vi "Request Events.vi"(8 "error in (no error)":errorcluster, 11 "VolatusAPI in":refnum<class "VolatusAPI.lvclass">) -> (0 "error out":errorcluster, 2 "Events":T1[](array[typedef]), 3 "VolatusAPI out":refnum<class "VolatusAPI.lvclass">)   [LabVIEW 2020, in "Volatus.lvlib" / "VolatusAPI.lvclass"]
uses:
  VolatusAPI.lvclass
  VolatusAPI.lvclass/VolatusAPI.ctl
  Event API/EventAPI.lvclass
  Event Level.ctl
  Volatus.lvlib
  Event.ctl
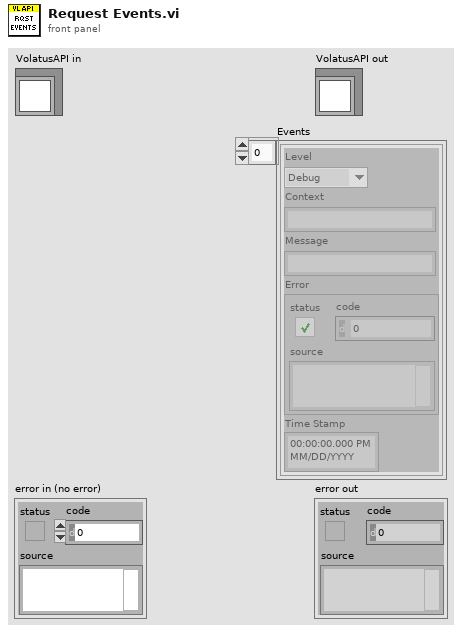
[diagram p1: front panel]
types:
  T1 = typedef "Volatus.lvlib/Event.ctl" = cluster{"Level":T2, "Context":string, "Message":string, "Error":errorcluster, "Time Stamp":timestamp}
  T2 = typedef "Volatus.lvlib/Event Level.ctl" = enum16{"Debug", "Info", "Warning", "Error"}
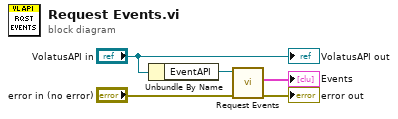
[diagram p0: block diagram]
diagram:
  n1 = Unbundle By Name("VolatusAPI in") -> ("EventAPI"=w4:refnum<class "EventAPI.lvclass">)
  n2 = call "Request Events.vi"("error in (no error)"="error in (no error)", "EventAPI in"=w4) -> ("error out"=→"error out":errorcluster, "Events"=→"Events":T1[])  [unwired: 7 in, 1 out]
  "VolatusAPI out" <- "VolatusAPI in"
